vi "xijk_load_from_file_choose_file.vi"(8 "error in":errorcluster, 10 "start path":path=path "", 11 "save cluster in":T1={{"axes in"={"min x-axis excitation"=0, "max x-axis excitation"=0, "min x-axis emission"=0, "max x-axis emission"=0, "precision of results"=2}, "plot colors in"={"Lanscape Portrait"=FALSE, "Plot logarithmic"=FALSE, "Ex/Em filters double"=FALSE, "Line colors"=[]}}, "search paths in"={"Paths"={"Path: Excitation filters"=path "", "Path: Dicroic filters"=path "", "Path: Emission filters"=path "", "Path reget"=path ""}, "table excitation"=[], "table dicroics"=[], "table emission"=[], "Integers"={"Select result number"=0}, "boolean selector array"=[], "table for calculation automagic"=[]}, "spectra parameters in"={"Booleans"={"Unknown detector"=FALSE, "Dual band filters"=FALSE, "Dual emission by cubes"=FALSE, "FRET"=FALSE}, "Integers"={"Light source"=0, "Number of fluorophores"=0, "Wavelength of laser (nm) 1"=0, "Broadness of laser (nm) 1"=0.0, "Wavelength of laser (nm) 2"=0, "Broadness of laser (nm) 2"=0.0, "Template"=0}, "Doubles"={"Molar extinction 1"=0.0, "Molar extinction 2"=0.0, "Quantum efficiency 1"=0.0, "Quantum efficiency 2"=0.0}}, "filepaths in"={"Excitation filter 1"=path "", "Dichroic filter 1"=path "", "Emission filter 1"=path "", "Excitation filter 2"=path "", "Dichroic filter 2"=path "", "Emission filter 2"=path "", "Extra em filter 1"=path "", "Extra em filter 2"=path "", "Light source file"=path "", "Fluorophore absorption 1"=path "", "Fluorophore emission 1"=path "", "Fluorophore absorption 2"=path "", "Fluorophore emission 2"=path "", "Detector"=path ""}} {"?"."axes in"."precision of results" max=8 step=1}) -> (0 "error out":errorcluster, 2 "path out":path caption="start path", 3 "save cluster out":T1={{"axes in"={"min x-axis excitation"=0, "max x-axis excitation"=0, "min x-axis emission"=0, "max x-axis emission"=0, "precision of results"=2}, "plot colors in"={"Lanscape Portrait"=FALSE, "Plot logarithmic"=FALSE, "Ex/Em filters double"=FALSE, "Line colors"=[]}}, "search paths in"={"Paths"={"Path: Excitation filters"=path "", "Path: Dicroic filters"=path "", "Path: Emission filters"=path "", "Path reget"=path ""}, "table excitation"=[], "table dicroics"=[], "table emission"=[], "Integers"={"Select result number"=0}, "boolean selector array"=[], "table for calculation automagic"=[]}, "spectra parameters in"={"Booleans"={"Unknown detector"=FALSE, "Dual band filters"=FALSE, "Dual emission by cubes"=FALSE, "FRET"=FALSE}, "Integers"={"Light source"=0, "Number of fluorophores"=0, "Wavelength of laser (nm) 1"=0, "Broadness of laser (nm) 1"=0.0, "Wavelength of laser (nm) 2"=0, "Broadness of laser (nm) 2"=0.0, "Template"=0}, "Doubles"={"Molar extinction 1"=0.0, "Molar extinction 2"=0.0, "Quantum efficiency 1"=0.0, "Quantum efficiency 2"=0.0}}, "filepaths in"={"Excitation filter 1"=path "", "Dichroic filter 1"=path "", "Emission filter 1"=path "", "Excitation filter 2"=path "", "Dichroic filter 2"=path "", "Emission filter 2"=path "", "Extra em filter 1"=path "", "Extra em filter 2"=path "", "Light source file"=path "", "Fluorophore absorption 1"=path "", "Fluorophore emission 1"=path "", "Fluorophore absorption 2"=path "", "Fluorophore emission 2"=path "", "Detector"=path ""}} {"?"."axes in"."precision of results" max=8 step=1})   [LabVIEW 2009]
uses:
  Type Def/save_cluster.ctl
  Type Def/axis_parameters.ctl
  Type Def/color_parameters.ctl
  Type Def/search_parameters.ctl
  Type Def/spectra_parameters.ctl
  Type Def/filepath.ctl
panel:
  # "Dichroic"
  # "Ex/Em filter"
  # "Fluorophore 1"
  # "Fluorophore 2"
  # "Laser /\nextra Em filter"
  # "Dichroic"
  # "Ex/Em filter"
  # "Fluorophore 1"
  # "Fluorophore 2"
  # "Laser /\nextra Em filter"
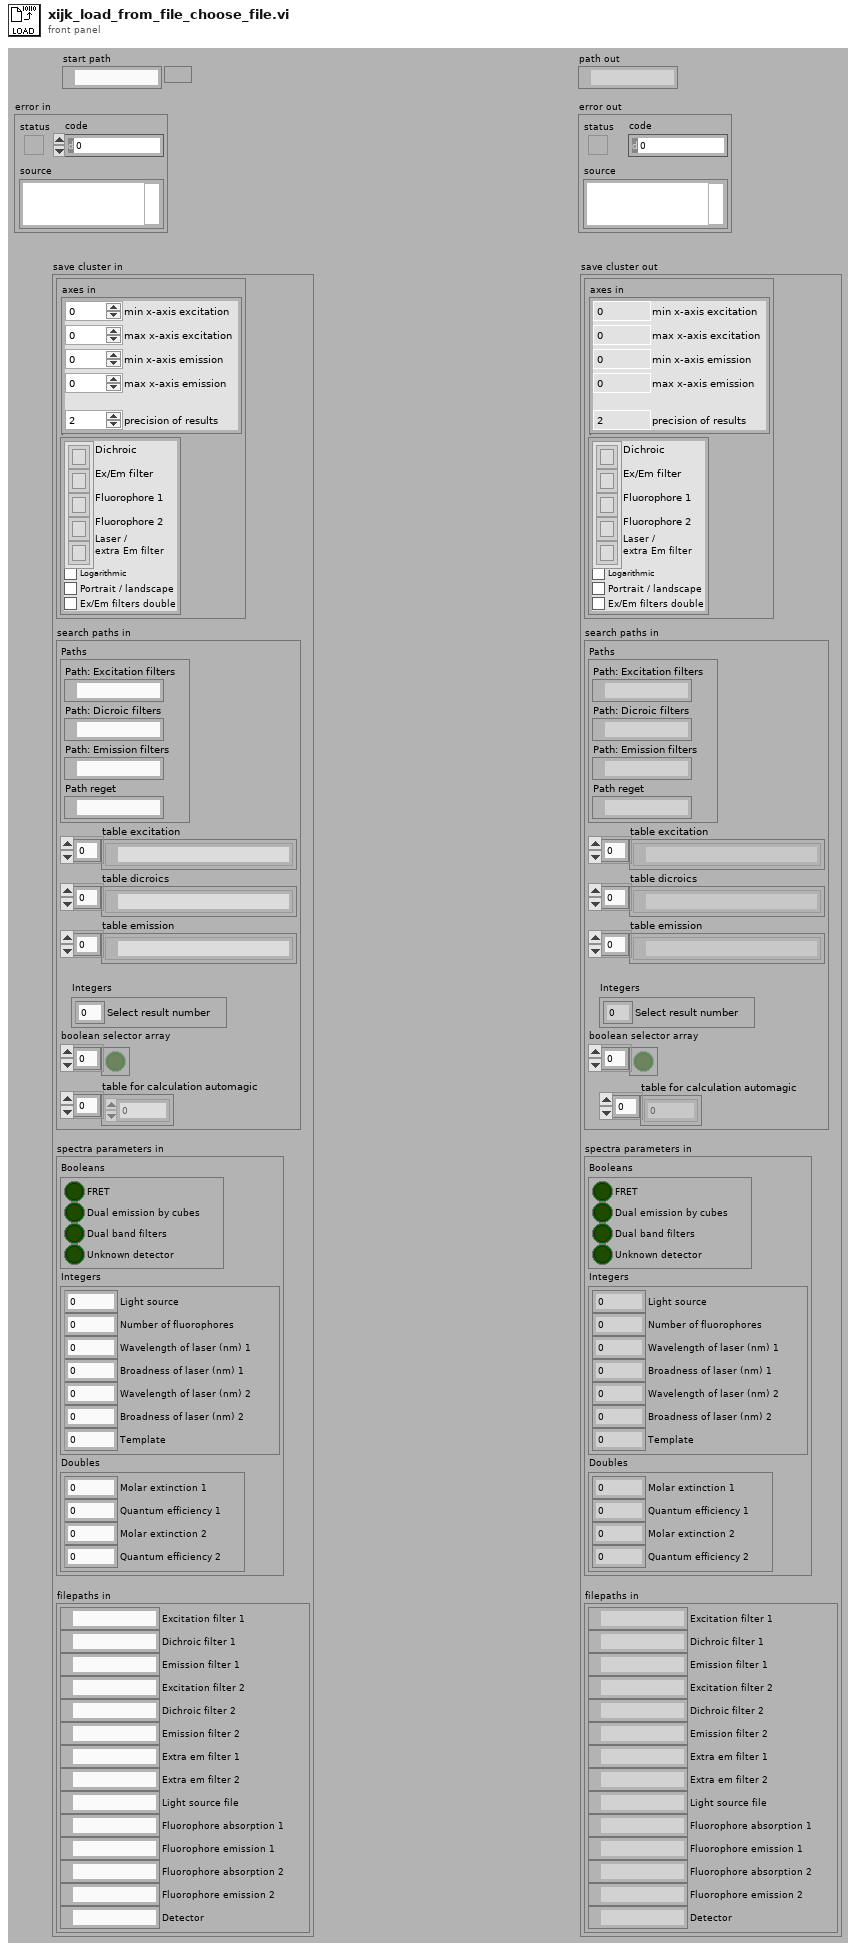
[diagram p1: front panel]
types:
  T1 = typedef "save_cluster.ctl" = cluster{cluster{"axes in":T2, "plot colors in":T3}, "search paths in":T4, "spectra parameters in":T5, "filepaths in":T6}
  T2 = typedef "axis_parameters.ctl" = cluster{"min x-axis excitation":u16, "max x-axis excitation":u16, "min x-axis emission":u16, "max x-axis emission":u16, "precision of results":u8}
  T3 = typedef "color_parameters.ctl" = cluster{"Lanscape Portrait":bool, "Plot logarithmic":bool, "Ex/Em filters double":bool, "Line colors":u32[]}
  T4 = typedef "search_parameters.ctl" = cluster{"Paths":cluster{"Path: Excitation filters":path, "Path: Dicroic filters":path, "Path: Emission filters":path, "Path reget":path}, "table excitation":path[], "table dicroics":path[], "table emission":path[], "Integers":cluster{"Select result number":u32}, "boolean selector array":bool[], "table for calculation automagic":i32[]}
  T5 = typedef "spectra_parameters.ctl" = cluster{"Booleans":cluster{"Unknown detector":bool, "Dual band filters":bool, "Dual emission by cubes":bool, "FRET":bool}, "Integers":cluster{"Light source":u16, "Number of fluorophores":u16, "Wavelength of laser (nm) 1":u16, "Broadness of laser (nm) 1":sgl, "Wavelength of laser (nm) 2":u16, "Broadness of laser (nm) 2":sgl, "Template":u16}, "Doubles":cluster{"Molar extinction 1":sgl, "Molar extinction 2":sgl, "Quantum efficiency 1":sgl, "Quantum efficiency 2":sgl}}
  T6 = typedef "filepath.ctl" = cluster{"Excitation filter 1":path, "Dichroic filter 1":path, "Emission filter 1":path, "Excitation filter 2":path, "Dichroic filter 2":path, "Emission filter 2":path, "Extra em filter 1":path, "Extra em filter 2":path, "Light source file":path, "Fluorophore absorption 1":path, "Fluorophore emission 1":path, "Fluorophore absorption 2":path, "Fluorophore emission 2":path, "Detector":path}
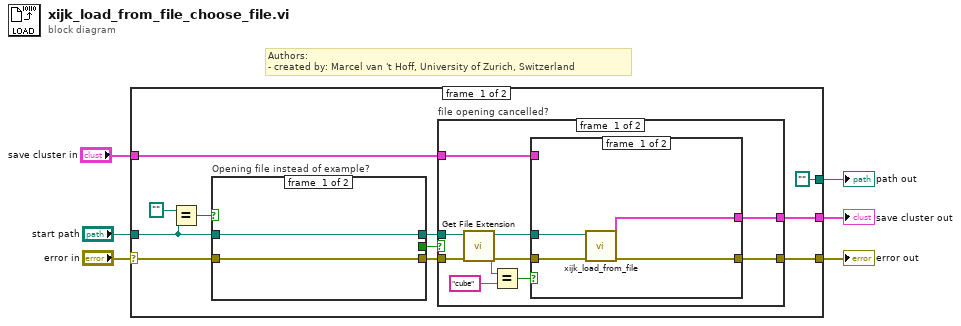
[diagram p0: block diagram]
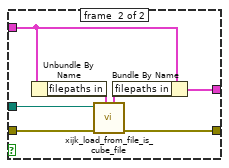
[diagram p2: hidden frame]
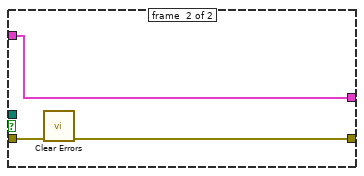
[diagram p3: hidden frame]
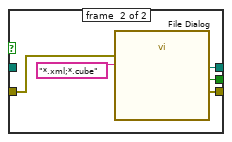
[diagram p4: hidden frame]
diagram:
  # "Authors: \n- created by: Marcel van 't Hoff, University of Zurich, Switzerland"
  n1 = case shown="No Error" "error in" {
    selector: "error in" -> [w15 w49]
    tunnel: [w17 w49] -> w6
    tunnel: "save cluster in" -> [w13 _]
    tunnel: [w12 _] -> w1
    tunnel: "start path" -> [w8 _]
    tunnel: [path "" _] -> w3
    frame #0 {
      n2 = Equal?(x=path "", y=w8) -> (x = y?=w10:bool)
      n3 = case "Opening file instead of example?" shown="False" w10 {
        tunnel: [w43 w47] -> w16
        tunnel: w15 -> [w42 w46]
        tunnel: [w42 w45] -> w14
        tunnel: w8 -> [w43 _]
        tunnel: [_ w44] -> w7
        frame #0 {
        }
        frame #1 {
          n4 = call "File Dialog"("error in"=w46, "pattern (all files)"="*.xml;*.cube") -> ("selected path"=w47:path, "cancelled"=w44:bool, "error out"=w45:errorcluster)  [unwired: 10 in, 1 out]
        }
      }
      n5 = case "file opening cancelled?" shown="False" w7 {
        tunnel: [w27 w39] -> w17
        tunnel: w16 -> [w21 _]
        tunnel: w14 -> [w20 w40]
        tunnel: w13 -> [w19 w41]
        tunnel: [w18 w41] -> w12
        frame #0 {
          n6 = call <vilib>:"Get File Extension.vi"("error in (no error)"=w20, "file"=w21) -> ("error out"=w26:errorcluster, "lowercase file extension"=w24:string, "dup file"=w25:path)  [unwired: 6 in, 1 out]
          n7 = Equal?(x=w24, y="cube") -> (x = y?=w22:bool)
          n8 = case shown="False" w22 {
            tunnel: [w31 w37] -> w27
            tunnel: w26 -> [w30 w38]
            tunnel: w25 -> [w29 w36]
            tunnel: w19 -> [_ w33]
            tunnel: [w28 w32] -> w18
            frame #0 {
              n9 = call "xijk_load_from_file.vi"("error in"=w30, "file path (dialog if empty)"=w29) -> ("error out"=w31:errorcluster, "load cluster out"=w28:T1)  [unwired: 8 in]
            }
            frame #1 {
              n10 = Unbundle By Name(w33) -> ("filepaths in"=w35:T6)
              n11 = call "xijk_load_from_file_is_cube_file.vi"("filepaths in"=w35, "error in"=w38, "file path in"=w36) -> ("error out"=w37:errorcluster, "filepaths out"=w34:T6)  [unwired: 7 in]
              n12 = Bundle By Name(cluster=w33, "filepaths in"=w34) -> (w32:T1)
            }
          }
        }
        frame #1 {
          n13 = call <vilib>:"Clear Errors.vi"("error in (no error)"=w40) -> ("error out"=w39:errorcluster)  [unwired: 6 in]
        }
      }
    }
    frame #1 {
    }
  }
  "error out" <- w6
  "path out" <- w3
  "save cluster out" <- w1
